vi "Remove UA Monitor.vi"(8 "error in (no error)":errorcluster, 9 "node IDs":T2, 10 "subscription ID in":T4, 11 "OPC UA client refnum in":T1) -> (0 "error out":errorcluster, 3 "OPC UA client refnum out":T1)   [LabVIEW 2024, in "OPCUA.lvlib"]
uses:
  <vilib>/OPCUA/controls/OPC UA Client Refnum.ctl
  <vilib>/OPCUA/controls/Subscription ID.ctl
  <vilib>/OPCUA/controls/NodeIds.ctl
  <vilib>/OPCUA/controls/NodeId.ctl
  OPCUA.lvlib
  <vilib>/OPCUA/NI OPC UA Client.lvlib
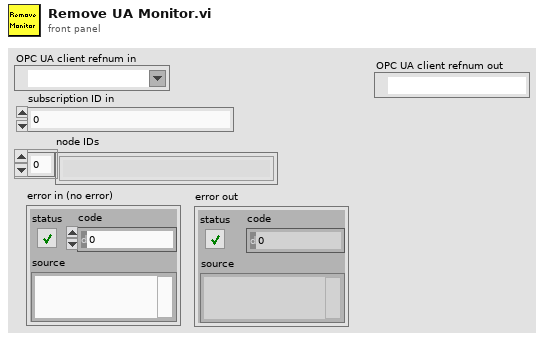
[diagram p1: front panel]
types:
  T1 = typedef "OPC UA Client Refnum.ctl" = refnum<k21>
  T2 = typedef "NodeIds.ctl" = T3[]
  T3 = typedef "NodeId.ctl" = string
  T4 = typedef "Subscription ID.ctl" = u32
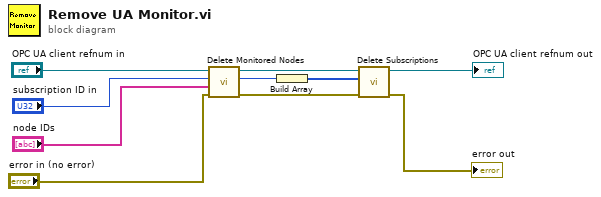
[diagram p0: block diagram]
diagram:
  n1 = call <vilib>:"Delete Monitored Nodes.vi"("error in (no error)"="error in (no error)", "node IDs"="node IDs", "subscription ID in"="subscription ID in", "OPC UA client refnum in"="OPC UA client refnum in") -> ("error out"=w6:errorcluster, "subscription ID out"=w2:T4, "OPC UA client refnum out"=w3:T1)  [unwired: 3 in, 2 out]
  n2 = Build Array(w2) -> (w1:T4[])
  n3 = call <vilib>:"Delete Subscriptions.vi"("error in (no error)"=w6, "subscription IDs"=w1, "OPC UA client refnum in"=w3) -> ("error out"=→"error out":errorcluster, "OPC UA client refnum out"=→"OPC UA client refnum out":T1)  [unwired: 6 in, 1 out]
